vi "Read Data.vi"(6 "chip select  (1st chip)":enum16{"1st chip", "2nd chip"}(ring), 8 "error in (no error)":errorcluster, 11 "LCD in":refnum<class "Character LCD.lvclass">) -> (0 "error out":errorcluster, 1 "data":u8=97 format="%.0x", 3 "LCD out":refnum<class "Character LCD.lvclass">)   [LabVIEW 2015, in "HD44780 Host.lvlib"]
uses:
  HD44780 Host.lvlib
  Internal/LCD Class/Character LCD.lvclass
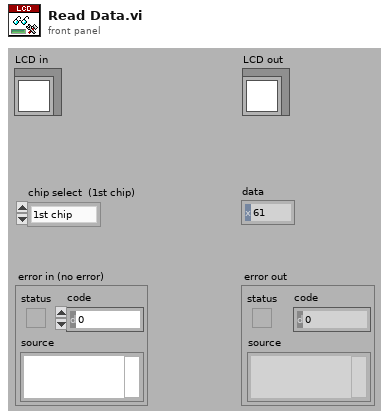
[diagram p1: front panel]
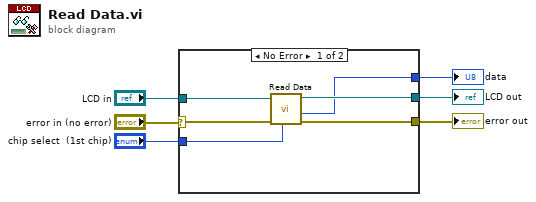
[diagram p0: block diagram]
diagram:
  n1 = case shown="No Error" "error in (no error)" {
    selector: "error in (no error)" -> [w8 w14]
    tunnel: "chip select  (1st chip)" -> [w12 _]
    tunnel: [w9 w14] -> w5
    tunnel: "LCD in" -> [w11 w13]
    tunnel: [w10 w13] -> w2
    tunnel: [w7 _] -> w1
    frame No Error {
      n2 = call-dynamic "Read Data.vi"("chip select  (1st chip)"=w12, "error in (no error)"=w8, "Character LCD in"=w11) -> ("error out"=w9:errorcluster, "data"=w7:u8, "Character LCD out"=w10:refnum<class "Character LCD.lvclass">)  [unwired: 6 in]
    }
    frame Error {
    }
  }
  "error out" <- w5
  "LCD out" <- w2
  "data" <- w1
